vi "Create App.vi"(9 "Alias":string, 10 "Actor":refnum<class "Actor.lvclass">) -> (0 "error out":errorcluster, 3 "Self Actor out":refnum<class "Self Actor.lvclass">)   [LabVIEW 2021, in "AAM.lvlib" / "Self Actor.lvclass"]
uses:
  Self Actor.lvclass
  Actor/Actor.lvclass
  Self Actor.lvclass/Self Actor.ctl
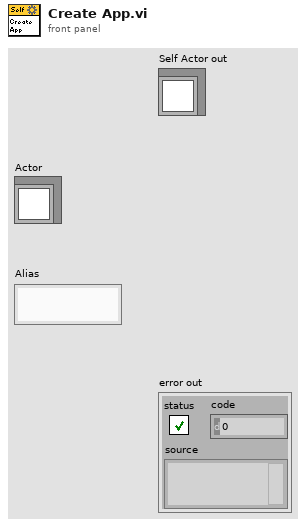
[diagram p1: front panel]
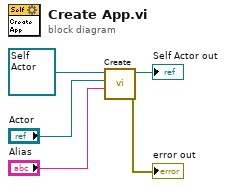
[diagram p0: block diagram]
diagram:
  n1 = call-dynamic "Create.vi"("Alias"="Alias", "Actor"="Actor", "Self Actor in"=refnum<class "Self Actor.lvclass"> refnum) -> ("error out"=→"error out":errorcluster, "Self Actor out"=→"Self Actor out":refnum<class "Self Actor.lvclass">)  [unwired: 7 in]
